vi "Qtegra_GetData.vi"() -> ()   [LabVIEW 2013]
panel:
  out "Waveform Chart":dbl(graph)
  out "data of detector":string
  in  "Command":string="GetData"
  in  "detector":string="H1_CDD"
  out "answer":string
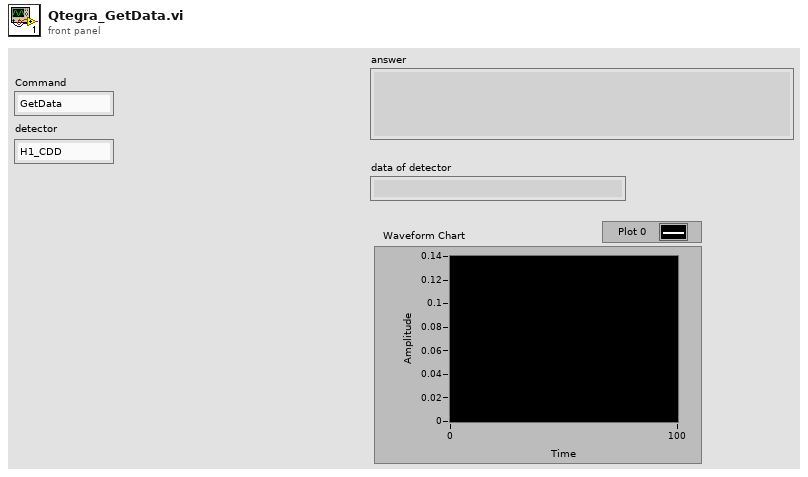
[diagram p1: front panel]
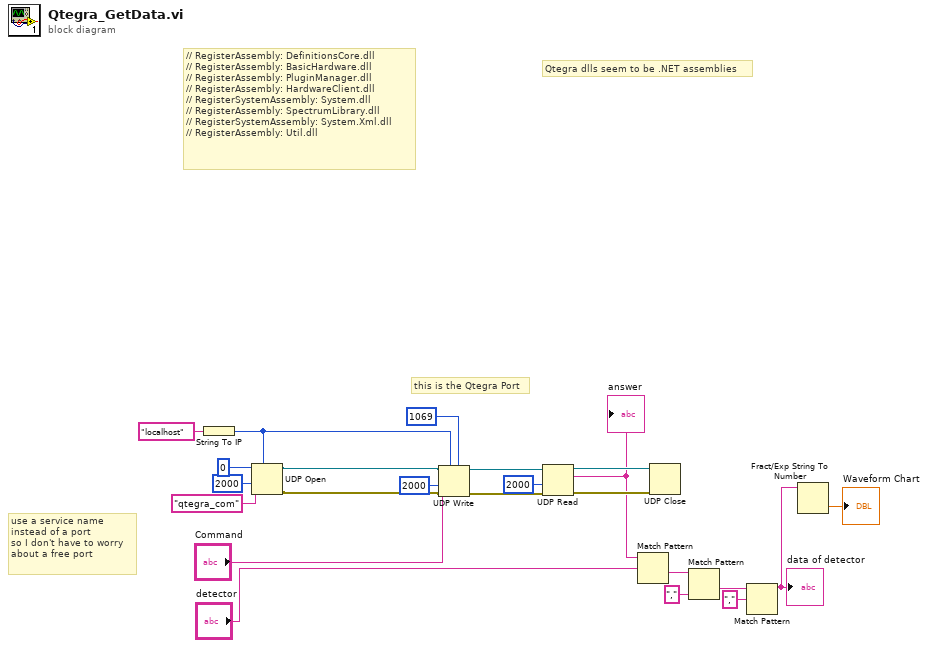
[diagram p0: block diagram]
diagram:
  # "use a service name\ninstead of a port\nso I don't have to worry\nabout a free port"
  # "this is the Qtegra Port"
  # "Qtegra dlls seem to be .NET assemblies"
  # "// RegisterAssembly: DefinitionsCore.dll\n// RegisterAssembly: BasicHardware.dll\n// RegisterAssembly: PluginManager.dll\n// RegisterAssembly: HardwareClient.dll\n// RegisterSystemAssembly: System.dll\n// RegisterAssembly: SpectrumLibrary.dll\n// RegisterSystemAssembly: System.Xml.dll\n// RegisterAssembly: Util.dll"
  n1 = String To IP(1:"localhost" ("name")) -> (0:w18:u32)
  n2 = UDP Open(7:w18, 9:2000 ("timeout ms (25000)"), 10:"qtegra_com" ("service name"), 11:u16 0 ("port")) -> (port=w20:refnum<k16>, 0:w19:errorcluster)  [unwired: 1 in, 1 out]
  n3 = UDP Write(address=w18, port or service name=u16 1069, connection ID=w20, data in="Command", 8:w19, 9:2000 ("timeout ms (25000)")) -> (error out=w15:errorcluster, 3:w16:refnum<k16>)
  n4 = UDP Read(connection ID=w16, timeout ms (25000)=2000, 8:w15) -> (data out=w8:string, error out=w10:errorcluster, 3:w11:refnum<k16>)  [unwired: 1 in, 2 out]
  "answer" <- w8
  n5 = Match Pattern(string=w8, regular expression="detector") -> (after substring=w6:string)  [unwired: 1 in, 3 out]
  n6 = UDP Close(connection ID=w11, 8:w10) -> ()  [unwired: 2 out]
  n7 = Match Pattern(string=w6, regular expression=",") -> (after substring=w4:string)  [unwired: 1 in, 3 out]
  n8 = Match Pattern(string=w4, regular expression=",") -> (before substring=w1:string)  [unwired: 1 in, 3 out]
  "data of detector" <- w1
  n9 = Fract/Exp String To Number(string=w1) -> (number=→"Waveform Chart":dbl)  [unwired: 3 in, 1 out]
